vi "FP_Read_Cap_Sensor.vi"() -> ()   [LabVIEW 2018, in "Tracker.lvlib"]
uses:
  Tracker.lvlib
  <vilib>/Utility/miscctls.llb/LVPointTypeDef.ctl
  <vilib>/Instr/_visa.llb/Select Event Type.ctl
  <vilib>/Instr/_visa.llb/VISA Open Access Mode.ctl
  <vilib>/Instr/_visa.llb/VISA Set IO Buffer Mask.ctl
  <vilib>/Instr/_visa.llb/VISA Configure Serial Port (Instr).vi
  <vilib>/ptbypt/NI_PtbyPt.lvlib
panel:
  out "TDMS file reference":refnum<k34>
  in  "Save file path":path
  out "VISA Fail":bool
  out "VISA OK":bool
  in  "Connect":bool
  in  "Less samples":bool
  in  "More samples":bool
  in  "Reset counter":bool
  out "Waveform Chart":cluster{i32, i16}(graph) caption="Waveform Chart - Dark"
  out "ms to read/samples":string
  out "N licks":i32
  out "error out":errorcluster
  in  "Threshold":i32=500
  in  "Stop":bool
  in  "VISA resource name":refnum<visa-resource-name>="COM10"
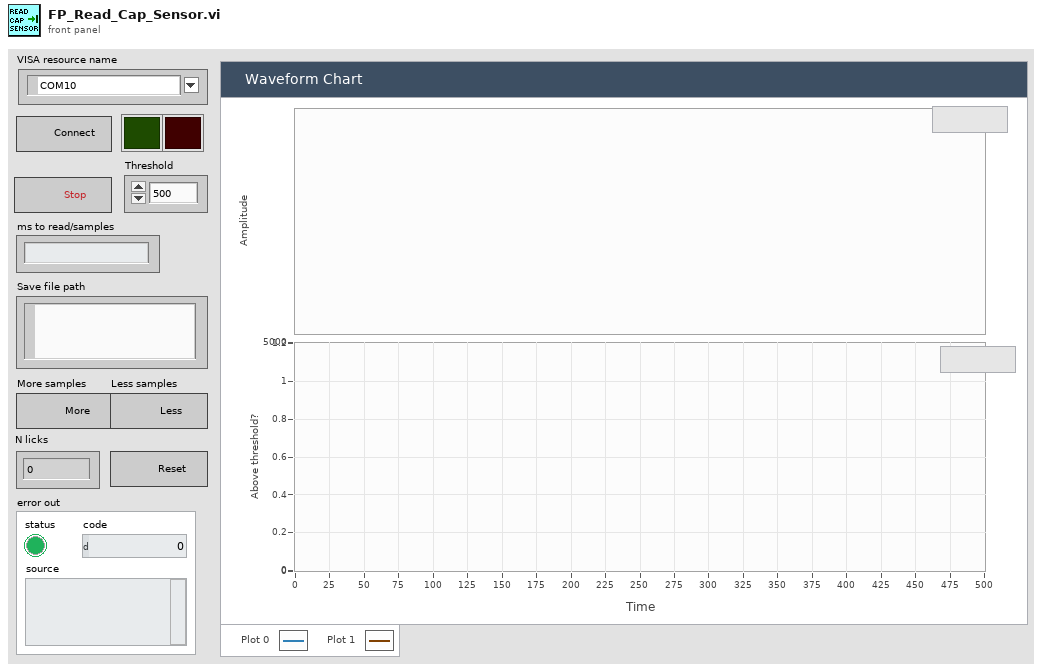
[diagram p1: front panel]
types:
  T1 = enum8{"Enabled", "Disabled", "Disabled and Grayed Out"}
  T2 = typedef "Select Event Type.ctl" = u32
  T3 = typedef "LVPointTypeDef.ctl" = cluster{"Horizontal":i16, "Vertical":i16}
  T4 = typedef "VISA Set IO Buffer Mask.ctl" = u16
  T5 = typedef "VISA Open Access Mode.ctl" = u32
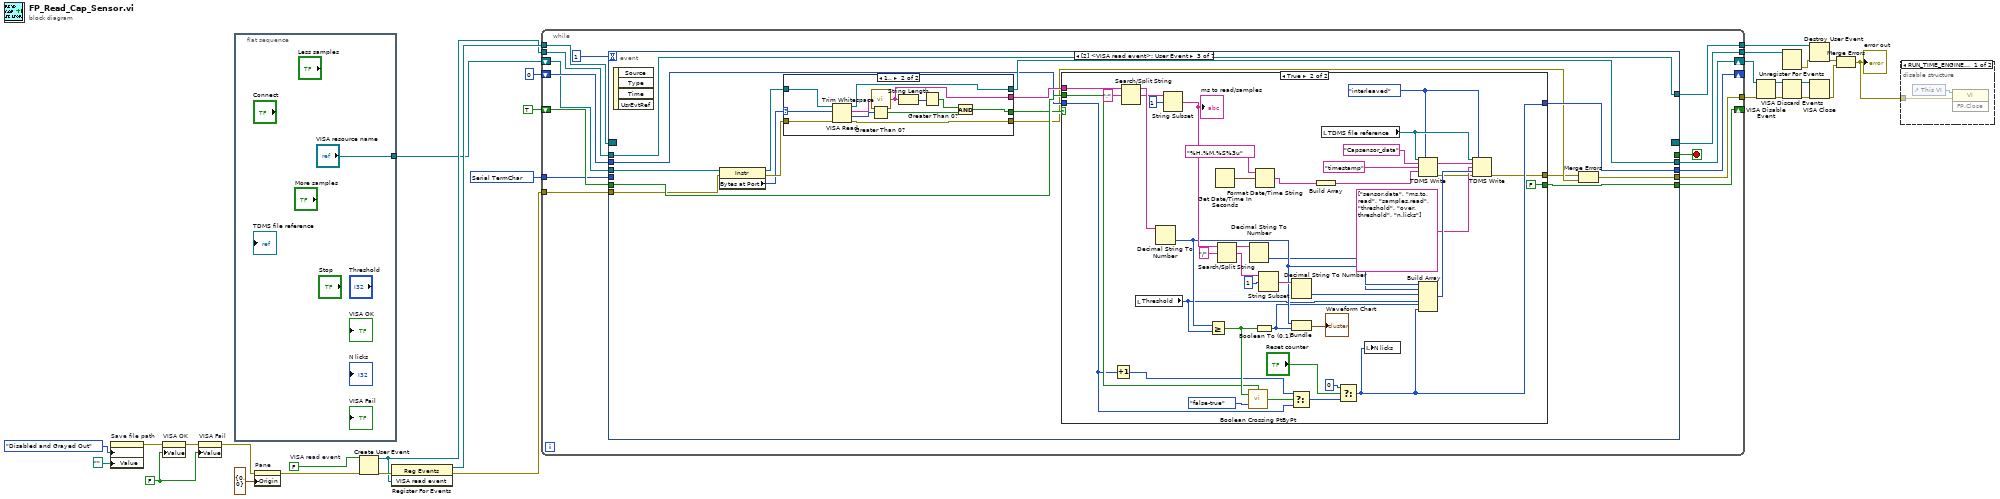
[diagram p0: block diagram]
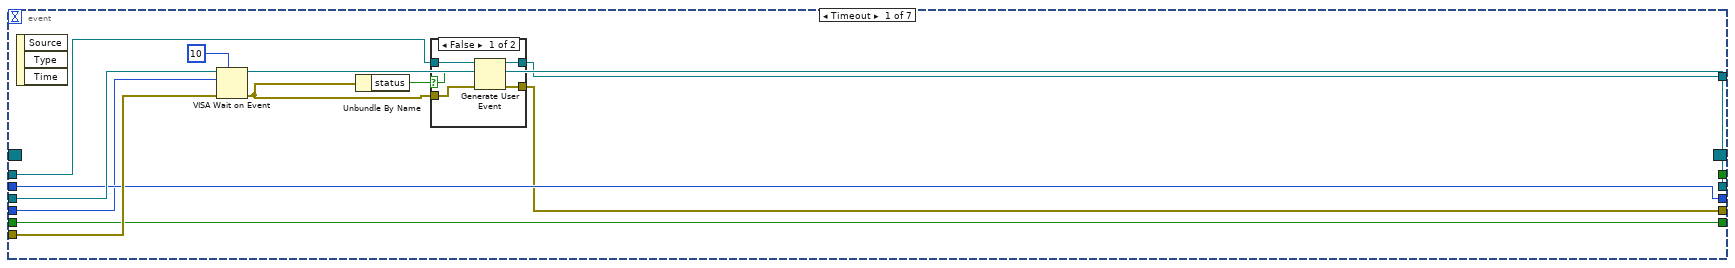
[diagram p3: hidden frame]
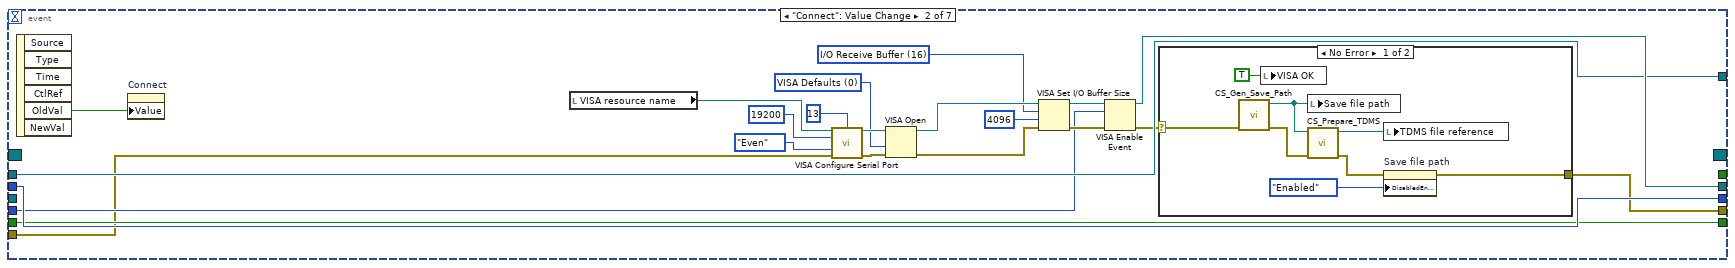
[diagram p5: hidden frame]
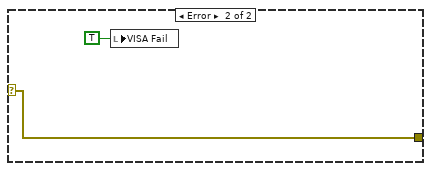
[diagram p6: hidden frame]
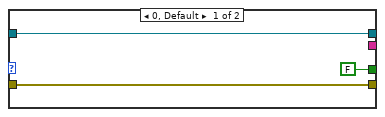
[diagram p8: hidden frame]
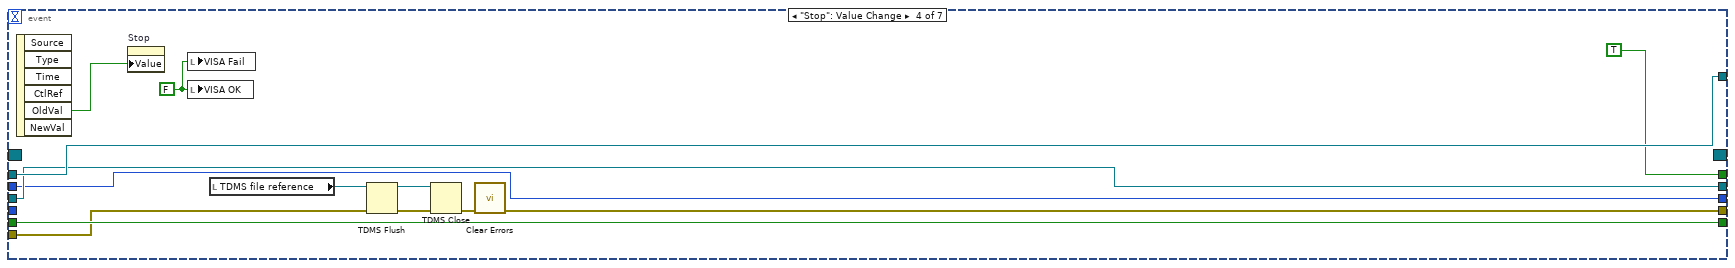
[diagram p9: hidden frame]
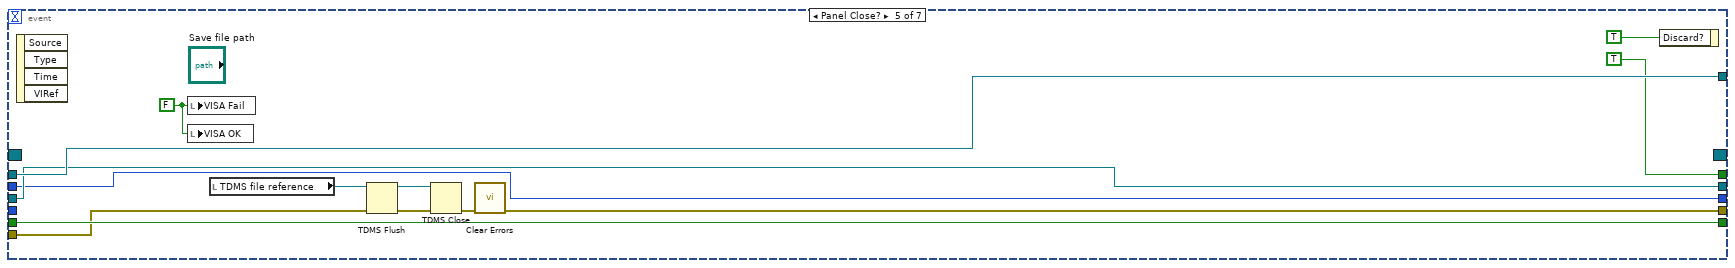
[diagram p10: hidden frame]
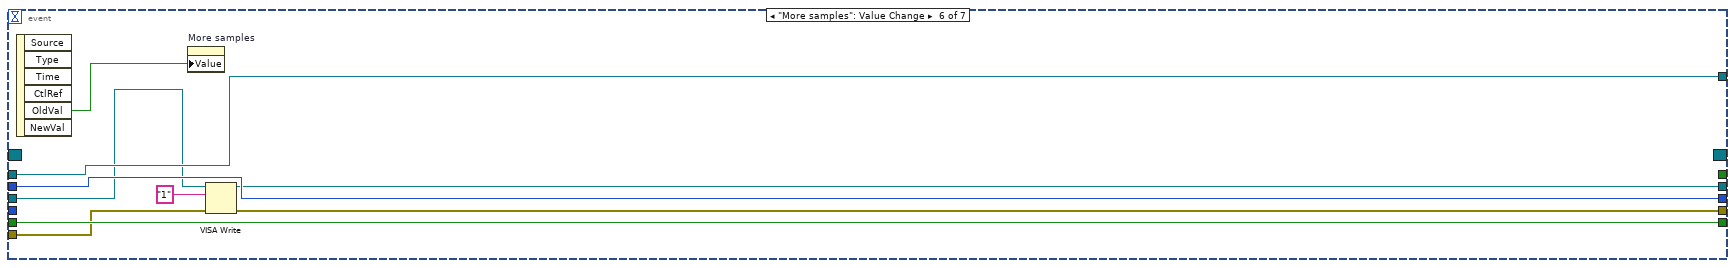
[diagram p11: hidden frame]
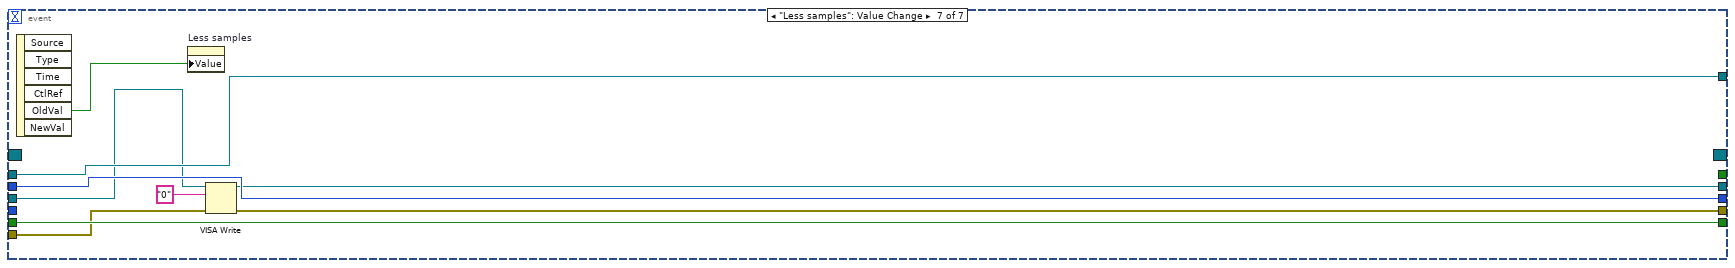
[diagram p12: hidden frame]
diagram:
  w7 = FALSE
  w8 = T2 1073684516 items=["Service Request"=1073684491, "Trigger"=3221168138, "Clear"=1073684493, "VXI Signal"=1073684512, "VXI/VME Interrupt"=3221168161, "VXI/VME Sysfail"=1073684509, "VXI/VME Sysreset"=1073684510, "GPIB CIC"=1073684498, "GPIB Talk"=1073684499, "GPIB Listen"=1073684500, "PXI Interrupt"=1073684514, "Serial Break"=1073684515, "Serial TermChar"=1073684516, "Serial CTS"=1073684521, "Serial DSR"=1073684522, "Serial DCD"=1073684524, "Serial RI"=1073684526, "Serial Character"=1073684533, "USB Interrupt"=1073684535, "All Enabled"=1073709055] ("Event Type")
  w22 = FALSE  # VISA read event
  n1 = property on="Save file path" class="Path"("DisabledEnum"=T1."Disabled and Grayed Out" ("Disabled"), "Value"=path "") -> (error out=w2:errorcluster)  [unwired: 2 in, 1 out]
  n2 = property on="VISA OK" class="Bool (strict)"(error in=w2, "Value"=w7) -> (error out=w6:errorcluster)  [unwired: 1 in, 1 out]
  n3 = property on="VISA Fail" class="Bool (strict)"(error in=w6, "Value"=w7) -> (error out=w5:errorcluster)  [unwired: 1 in, 1 out]
  n4 = flat-sequence {
    tunnel: ["VISA resource name"] -> w11
    frame #0 {
    }
  }
  n5 = property on="Pane" class="Pane"(error in=w5, "Origin"=T3 {"Horizontal"=0, "Vertical"=0}) -> (error out=w10:errorcluster)  [unwired: 1 in, 1 out]
  n6 = Create User Event(user event datatype=w22, error in=w10) -> (user event=w15:refnum<user-event>, error out=w21:errorcluster)
  n7 = register-events(error in=w21, w15) -> (reference out=w20:refnum<event-registration>, error out=w12:errorcluster)  [unwired: 1 in]
  n8 = while {
    shift-right: [w43] -> _
    shift-left: 0 -> [w44]
    shift-right: [w42] -> _
    shift-left: TRUE -> [w45]
    tunnel: w20 -> [w41]
    tunnel: w12 -> [w40]
    tunnel: [w38] -> w19
    tunnel: [w37] -> w18
    tunnel: w15 -> [w36]
    tunnel: [w35] -> w14
    shift-right: [w32] -> w9
    shift-left: w11 -> [w39]
    tunnel: w8 -> [w31]
    stop <- w33 stop-if-true
    n9 = event shown="[2] <VISA read event>: User Event" {
      selector: w41 -> [_ _ _ _ _ _ _]
      dyn-events: [_ _ _ _ _ _ _] -> w37
      timeout: 1 -> [_ _ _ _ _ _ _]
      tunnel: [w54 w72 w112 w181 w194 w199 w208] -> w32
      tunnel: w45 -> [w52 w69 w107 w179 w192 w202 w211]
      tunnel: w44 -> [w53 w71 w106 w180 w193 w203 w212]
      tunnel: [w53 w71 w105 w180 w193 w203 w212] -> w43
      tunnel: [w52 w69 w103 w179 w192 w202 w211] -> w42
      tunnel: w40 -> [w56 w65 w102 w173 w186 w197 w206]
      tunnel: w39 -> [w55 _ w101 w181 w194 w200 w209]
      tunnel: [w47 w66 w98 w170 w183 w196 w205] -> w38
      tunnel: w36 -> [w49 w70 w99 w182 w195 w204 w213]
      tunnel: [w48 w70 w99 w182 w195 w204 w213] -> w35
      tunnel: [_ _ _ TRUE TRUE _ _] -> w33
      tunnel: w31 -> [w46 w68 _ _ _ _ _]
      event Timeout {
        n10 = event-data() -> ()  [unwired: 1 in, 3 out]
        n11 = VISA Wait on Event(7:u32 10 ("timeout (0)"), 8:w56, 10:w46, 11:w55) -> (0:w50:errorcluster, 3:w54:refnum<visa-resource-name>)  [unwired: 1 in, 2 out]
        n12 = Unbundle By Name(w50) -> ("status"=w51:bool)
        n13 = case shown="False" w51 {
          selector: w51 -> [w61 _]
          tunnel: w50 -> [w62 w63]
          tunnel: w49 -> [w60 w64]
          tunnel: [w59 w64] -> w48
          tunnel: [w58 w63] -> w47
          frame False {
            n14 = Generate User Event(user event=w60, event data cluster=w61, error in=w62) -> (user event out=w59:refnum<user-event>, error out=w58:errorcluster)  [unwired: 1 in]
          }
          frame True {
          }
        }
      }
      event "Connect": Value Change {
        w78 = T4 16 items=["I/O Receive Buffer"=16, "I/O Transmit Buffer"=32, "I/O Receive and Transmit Buffer"=48] ("Mask")
        w74 = T5 0 items=["VISA Defaults"=0, "Exclusive Lock"=1, "Load Configured Settings"=4] ("Access Mode")
        n15 = event-data() -> ("OldVal"=w86:bool)  [unwired: 1 in, 5 out]
        n16 = property on="Connect" class="Bool (strict)"("Value"=w86) -> ()  [unwired: 2 in, 2 out]
        n17 = local read "VISA resource name"() -> (w73:refnum<visa-resource-name>)
        n18 = call-poly "VISA Configure Serial Port"("VISA resource name"=w73, "termination char\n(0xA = '\\n' = LF)"=u8 13 ("termination char\n(0xA = '\\n' = LF)"), "baud rate (9600)"=u32 19200, "parity (0:none)"=enum16{"None", "Odd", "Even", "Mark", "Space"}."Even", "error in (no error)"=w65) -> ("VISA resource name out"=w80:refnum<visa-resource-name>, "error out"=w81:errorcluster)  [unwired: 9 in]
        n19 = VISA Open(access mode=w74, error in (no error)=w81, VISA resource name=w80) -> (VISA resource name=w82:refnum<visa-resource-name>, error out=w83:errorcluster)  [unwired: 2 in]
        n20 = VISA Set I/O Buffer Size(VISA resource name=w82, mask (16)=w78, size (4096)=u32 4096, error in (no error)=w83) -> (VISA resource name out=w84:refnum<visa-resource-name>, error out=w85:errorcluster)
        n21 = VISA Enable Event(8:w85, 10:w68, 11:w84) -> (0:w67:errorcluster, 3:w72:refnum<visa-resource-name>)  [unwired: 1 in]
        n22 = case shown="No Error" w67 {
          selector: w67 -> [w89 w96]
          tunnel: [w93 w96] -> w66
          frame No Error {
            n23 = call "CS_Gen_Save_Path.vi"("error in (no error)"=w89) -> ("Error Out"=w88:errorcluster, "Save path"=w90:path)  [unwired: 9 in]
            n24 = local write "VISA OK"(TRUE ("VISA OK")) -> ()
            n25 = local write "Save file path"(w90) -> ()
            n26 = call "CS_Prepare_TDMS.vi"("error in (no error)"=w88, "Save path"=w90) -> ("error out"=w87:errorcluster, "Refnum out"=w91:refnum<k34>)  [unwired: 8 in]
            n27 = local write "TDMS file reference"(w91) -> ()
            n28 = property on="Save file path" class="Path"(error in=w87, "DisabledEnum"=T1."Enabled" ("Disabled")) -> (error out=w93:errorcluster)  [unwired: 1 in, 1 out]
          }
          frame Error {
            n29 = local write "VISA Fail"(TRUE ("VISA Fail")) -> ()
          }
        }
      }
      event User Event {
        n30 = event-data() -> ()  [unwired: 1 in, 4 out]
        n31 = property class="Instr"(reference=w101, error in=w102) -> (reference out=w110:refnum<visa-resource-name>, error out=w111:errorcluster, "Bytes at Port"=w108:u32)
        n32 = case shown="1.." w108 {
          selector: w108 -> [_ w159]
          tunnel: [w157 w169] -> w112
          tunnel: w111 -> [w155 w168]
          tunnel: w110 -> [w157 w167]
          tunnel: [FALSE w161] -> w104
          tunnel: [_ w160] -> w109
          tunnel: [w155 w158] -> w100
          frame 0, Default {
          }
          frame 1.. {
            n33 = VISA Read(VISA resource name=w167, byte count=w159, error in (no error)=w168) -> (VISA resource name out=w169:refnum<visa-resource-name>, read buffer=w165:string, return count=w166:u32, error out=w158:errorcluster)
            n34 = Greater Than 0?(x=w166) -> (x > 0?=w162:bool)
            n35 = call <vilib>:"Trim Whitespace.vi"("string"=w165) -> ("trimmed string"=w160:string)  [unwired: 1 in]
            n36 = String Length(string=w160) -> (length=w164:i32)
            n37 = Greater Than 0?(x=w164) -> (x > 0?=w163:bool)
            n38 = And(x=w163, y=w162) -> (x .and. y?=w161:bool)
          }
        }
        n39 = case shown="True" w104 {
          tunnel: w109 -> [_ w143]
          tunnel: w107 -> [_ w153]
          tunnel: w106 -> [w113 w145]
          tunnel: [w113 w126] -> w105
          tunnel: [_ FALSE] -> w103
          tunnel: [_ w124] -> w97
          frame False {
          }
          frame True {
            w122 = enum16{"decimated", "interleaved"}."interleaved" ("data layout (0:decimated)")
            n40 = Increment(x=w145) -> (x+1=w144:i32)
            n41 = Search/Split String(string=w143, search string/char (-)=";") -> (substring before match=w141:string, match + rest of string=w140:string)  [unwired: 1 in, 1 out]
            n42 = local read "Threshold"() -> (w128:i32)
            n43 = Decimal String To Number(string=w141) -> (number=w131:i32)  [unwired: 2 in, 1 out]
            n44 = String Subset(string=w140, offset (0)=1) -> (substring=w138:string)  [unwired: 1 in]
            "ms to read/samples" <- w138
            n45 = Greater Or Equal?(x=w131, y=w128) -> (x >= y?=w154:bool)
            n46 = Get Date/Time In Seconds() -> (seconds since 1Jan1904=w116:timestamp)
            n47 = Search/Split String(string=w138, search string/char (-)="/") -> (substring before match=w134:string, match + rest of string=w135:string)  [unwired: 1 in, 1 out]
            n48 = call <vilib>:"Boolean Crossing PtByPt.vi"("initialize"=w153, "direction"=enum16{"either", "false-true", "true-false"}."false-true", "input"=w154) -> ("crossing"=w151:bool)
            n49 = Decimal String To Number(string=w134) -> (number=w130:i32)  [unwired: 2 in, 1 out]
            n50 = Boolean To (0,1)(Boolean=w154) -> (0, 1=w127:i16)
            n51 = Format Date/Time String(time format string (%c)="%H.%M.%S%3u", seconds (now)=w116) -> (date/time string=w115:string)  [unwired: 1 in]
            n52 = String Subset(string=w135, offset (0)=1) -> (substring=w133:string)  [unwired: 1 in]
            n53 = Select(t=w144, s=w151, f=w145) -> (s? t:f=w149:i32)
            n54 = Decimal String To Number(string=w133) -> (number=w129:i32)  [unwired: 2 in, 1 out]
            n55 = Bundle(w131, w127) -> (→"Waveform Chart":cluster{i32, i16})  [unwired: 1 in]
            n56 = Build Array(w115) -> (w117:string[])
            n57 = local read "TDMS file reference"() -> (w123:refnum<k34>)
            n58 = Select(t=0, s="Reset counter", f=w149) -> (s? t:f=w126:i32)
            n59 = local write "N licks"(w126) -> ()
            n60 = TDMS Write(0:w123, 1:w122, 5:"Capsensor_data" ("group name"), 7:"timestamp", 9:w117) -> (6:w120:string, 15:w119:errorcluster)  [unwired: 1 in, 2 out]
            n61 = Build Array(w131, w130, w129, w128, w127, w126) -> (w132:i32[])
            n62 = TDMS Write(0:w123, 1:w122, 5:w120, 7:string[] ["sensor.data", "ms.to.read", "samples.read", "threshold", "over.threshold", "n.licks"] ("Columns Names"), 9:w132, 11:w119) -> (15:w124:errorcluster)  [unwired: 3 out]
          }
        }
        n63 = Merge Errors(w97, w100) -> (w98:errorcluster)
      }
      event "Stop": Value Change {
        w176 = FALSE
        n64 = event-data() -> ("OldVal"=w177:bool)  [unwired: 1 in, 5 out]
        n65 = property on="Stop" class="Bool (strict)"("Value"=w177) -> ()  [unwired: 2 in, 2 out]
        n66 = local write "VISA Fail"(w176) -> ()
        n67 = local write "VISA OK"(w176) -> ()
        n68 = local read "TDMS file reference"() -> (w175:refnum<k34>)
        n69 = TDMS Flush(4:w173, 7:w175) -> (0:w172:errorcluster, 3:w174:refnum<k34>)
        n70 = TDMS Close(8:w172, 11:w174) -> (0:w171:errorcluster)  [unwired: 1 out]
        n71 = call <vilib>:"Clear Errors.vi"("error in (no error)"=w171) -> ("error out"=w170:errorcluster)  [unwired: 5 in, 1 out]
      }
      event Panel Close? {
        w190 = FALSE
        n72 = event-data() -> ()  [unwired: 1 in, 4 out]
        n73 = local write "VISA Fail"(w190) -> ()
        n74 = local write "VISA OK"(w190) -> ()
        n75 = local read "TDMS file reference"() -> (w188:refnum<k34>)
        n76 = TDMS Flush(4:w186, 7:w188) -> (0:w185:errorcluster, 3:w187:refnum<k34>)
        n77 = TDMS Close(8:w185, 11:w187) -> (0:w184:errorcluster)  [unwired: 1 out]
        n78 = call <vilib>:"Clear Errors.vi"("error in (no error)"=w184) -> ("error out"=w183:errorcluster)  [unwired: 5 in, 1 out]
        n79 = event-data("Discard?"=TRUE) -> ()  [unwired: 1 in, 1 out]
      }
      event "More samples": Value Change {
        n80 = event-data() -> ("OldVal"=w201:bool)  [unwired: 1 in, 5 out]
        n81 = property on="More samples" class="Bool (strict)"("Value"=w201) -> ()  [unwired: 2 in, 2 out]
        n82 = VISA Write(VISA resource name=w200, write buffer="1", error in (no error)=w197) -> (VISA resource name out=w199:refnum<visa-resource-name>, error out=w196:errorcluster)  [unwired: 1 out]
      }
      event "Less samples": Value Change {
        n83 = event-data() -> ("OldVal"=w210:bool)  [unwired: 1 in, 5 out]
        n84 = property on="Less samples" class="Bool (strict)"("Value"=w210) -> ()  [unwired: 2 in, 2 out]
        n85 = VISA Write(VISA resource name=w209, write buffer="0", error in (no error)=w206) -> (VISA resource name out=w208:refnum<visa-resource-name>, error out=w205:errorcluster)  [unwired: 1 out]
      }
    }
  }
  n86 = VISA Disable Event(8:w19, 11:w9) -> (0:w27:errorcluster, 3:w29:refnum<visa-resource-name>)  [unwired: 2 in]
  n87 = Unregister For Events(event registration refnum=w18) -> (error out=w17:errorcluster)  [unwired: 1 in]
  n88 = VISA Discard Events(8:w27, 11:w29) -> (0:w26:errorcluster, 3:w28:refnum<visa-resource-name>)  [unwired: 2 in]
  n89 = Destroy User Event(user event=w14, error in=w17) -> (error out=w16:errorcluster)
  n90 = VISA Close(VISA resource name=w28, error in (no error)=w26) -> (error out=w25:errorcluster)
  n91 = Merge Errors(w16, w25) -> (w4:errorcluster)
  "error out" <- w4
  n92 = disable-structure shown="RUN_TIME_ENGINE==True" {
    disable-tunnel: w4 -> [w214 _]
    frame condition #0 {
      n93 = control-ref of="This VI"() -> (w215:refnum<vi>)
      n94 = invoke class="VI" method="FP.Close"(reference=w215, error in=w214) -> ()  [unwired: 1 in, 3 out]
    }
    frame condition #1 (active) {
    }
  }
